vi "All.vi"() -> ()   [LabVIEW 2020]
uses:
  <vilib>/vision/driver/IMAQdx.llb/IMAQdx Buffer Number Mode.ctl
  <vilib>/vision/driver/NI_Vision_Acquisition_Software.lvlib
  <resource>/objmgr/imaqdx.rc
panel:
  out "data out":string
  out "y":dbl
  out "x":dbl
  in  "Server Closed":string="The server VI closed the connection."
  in  "Number of Images":u32=10
  in  "Camera Name":refnum<k21> caption="IMAQdx Session"
  in  "Stop":bool
  out "Processing Frame Rate":dbl
  out "Images Missed":u32
  out "Start Image":T1(plugin-control)
  out "Threshold  Image":T1(plugin-control)
  out "Fill Holes  Image":T1(plugin-control)
  in  "Green":cluster{"Lower value":i32, "Upper value":i32}={"Lower value"=168, "Upper value"=255} {"Lower value" scale=0.0..255.0; "Upper value" scale=0.0..255.0}
  in  "Blue":cluster{"Lower value":i32, "Upper value":i32}={"Lower value"=148, "Upper value"=255} {"Lower value" scale=0.0..255.0; "Upper value" scale=0.0..255.0}
  in  "Red":cluster{"Lower value":i32, "Upper value":i32}={"Lower value"=158, "Upper value"=255} {"Lower value" scale=0.0..255.0; "Upper value" scale=0.0..255.0}
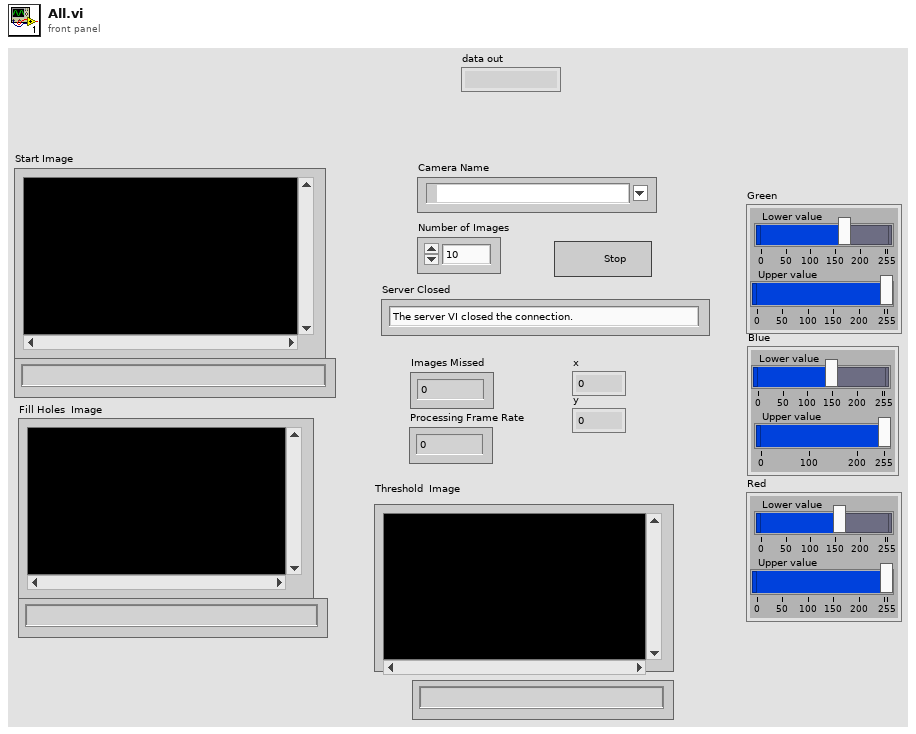
[diagram p1: front panel]
types:
  T1 = typedef "IMAQ Image.ctl" = refnum<image>
  T2 = typedef "IMAQdx.ctl" = refnum<k21>
  T3 = typedef "NI_Vision_Acquisition_Software.lvlib/IMAQdx Buffer Number Mode.ctl" = enum32{"Next", "Last", "Buffer Number", "Every", "Last New"}
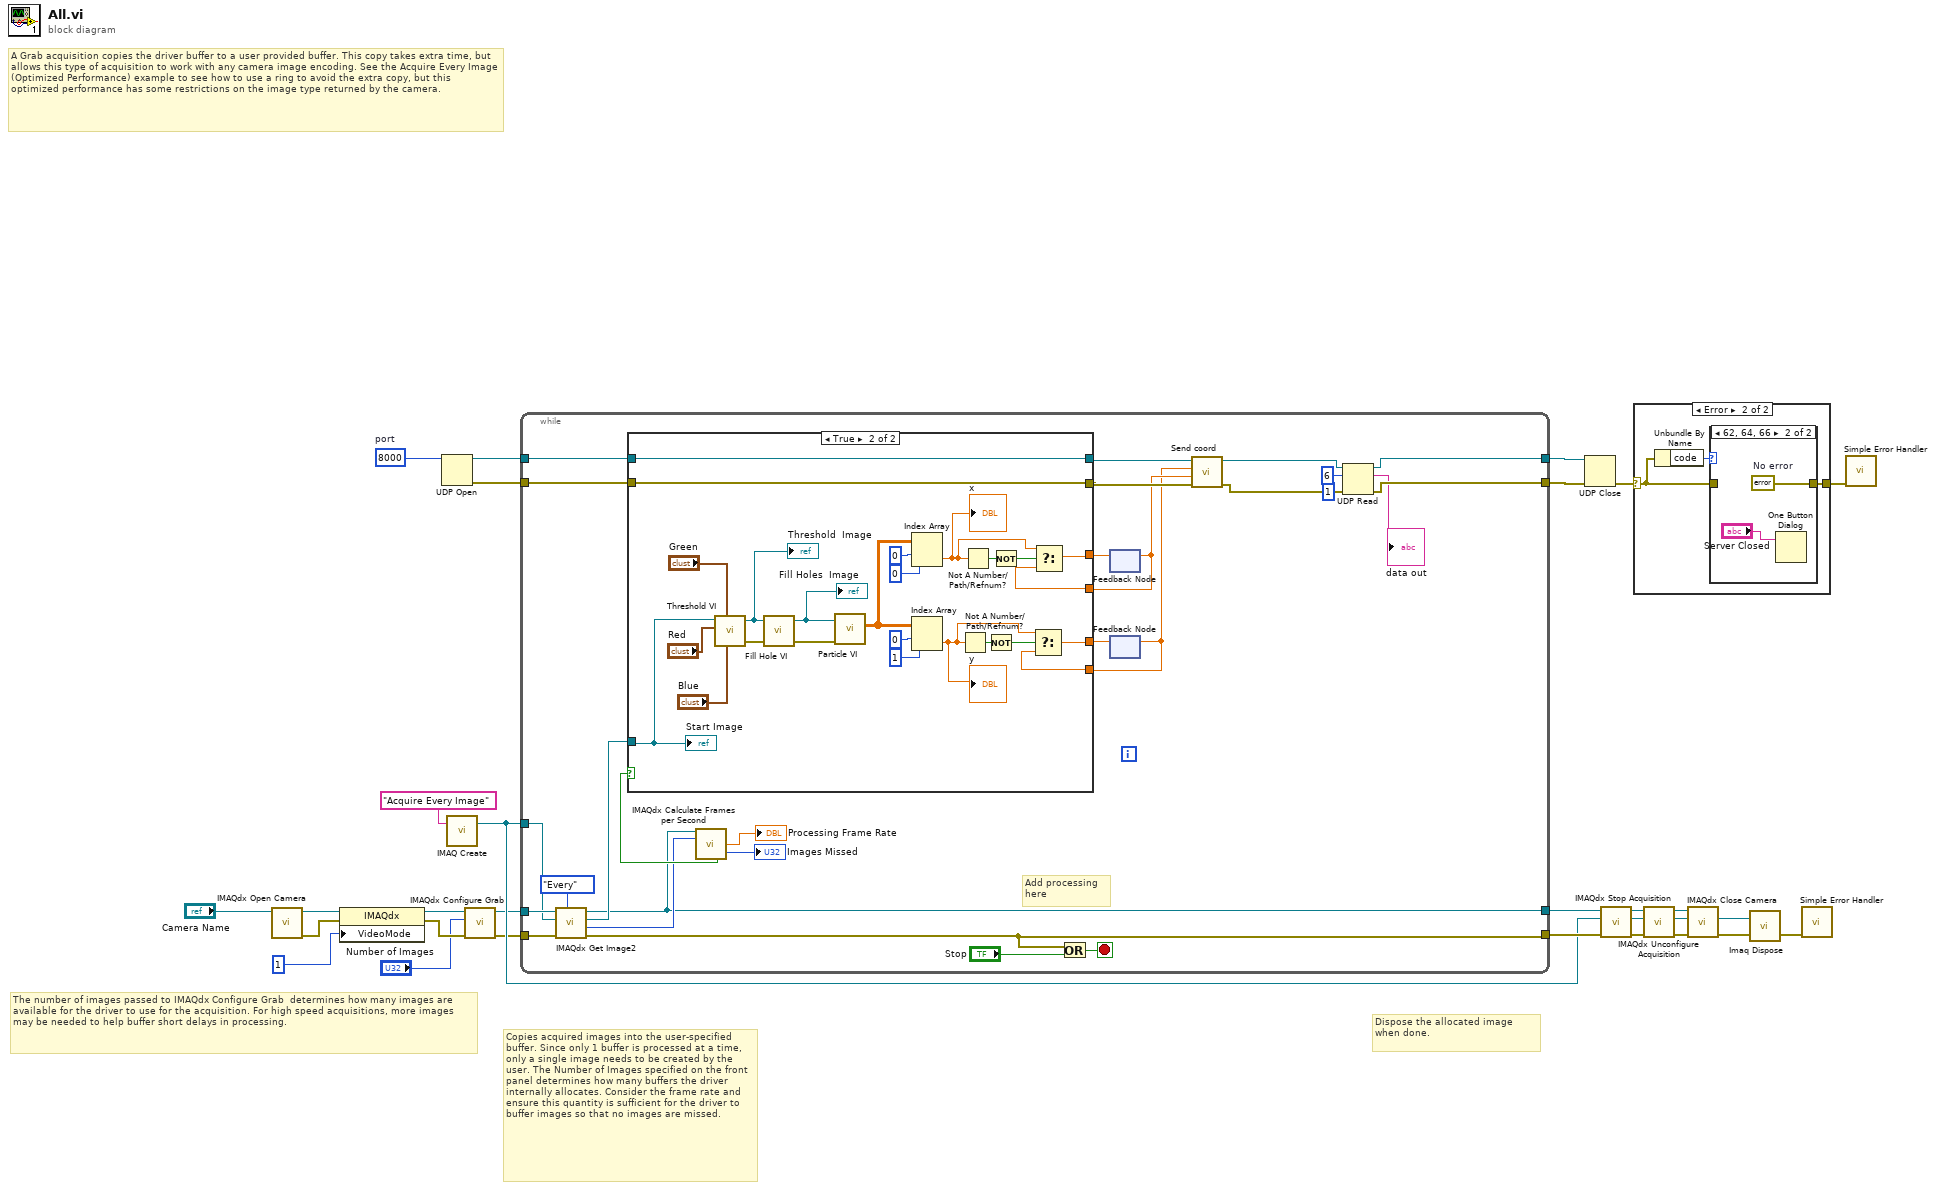
[diagram p0: block diagram]
diagram:
  w1 = u16 8000  # port
  # "The number of images passed to IMAQdx Configure Grab  determines how many images are available for the driver to use for the acquisition. For high speed acquisitions, more images may be needed to help buffer short delays in processing."
  # "Dispose the allocated image when done."
  # "A Grab acquisition copies the driver buffer to a user provided buffer. This copy takes extra time, but allows this type of acquisition to work with any camera image encoding. See the Acquire Every Image (Optimized Performance) example to see how to use a ring to avoid the extra copy, but this optimized performance has some restrictions on the image type returned by the camera."
  # "Copies acquired images into the user-specified buffer. Since only 1 buffer is processed at a time, only a single image needs to be created by the user. The Number of Images specified on the front panel determines how many buffers the driver internally allocates. Consider the frame rate and ensure this quantity is sufficient for the driver to buffer images so that no images are missed."
  n1 = call <vilib>:"IMAQdx Open Camera.vi"("Session In"="Camera Name") -> ("error out"=w18:errorcluster, "Session Out"=w19:T2)  [unwired: 2 in, 7 out]
  n2 = property class="IMAQdx"(reference=w19, error in=w18, "VideoMode"=u32 1) -> (reference out=w11:T2, error out=w10:errorcluster)
  n3 = UDP Open(11:w1) -> (port=w8:refnum<k16>, 0:w7:errorcluster)  [unwired: 4 in, 1 out]
  n4 = call "IMAQ Create"("Image Name"="Acquire Every Image") -> ("New Image"=w14:T1)  [unwired: 3 in, 2 out]
  n5 = call <vilib>:"IMAQdx Configure Grab.vi"("error in"=w10, "Number of Buffers"="Number of Images", "Session In"=w11) -> ("error out"=w12:errorcluster, "Session Out"=w13:T2)  [unwired: 7 in]
  n6 = while {
    tunnel: [w45] -> w16
    tunnel: w12 -> [w51]
    tunnel: w13 -> [w50]
    tunnel: [w34] -> w15
    tunnel: w14 -> [w48]
    tunnel: w8 -> [w43]
    tunnel: w7 -> [w42]
    tunnel: [w28] -> w4
    tunnel: [w29] -> w3
    stop <- w35 stop-if-true
    # "Avoid image display when falling behind."
    # "Add processing here"
    n7 = call <vilib>:"IMAQdx Get Image2.vi"("Buffer Number Mode (Next)"=IMAQdx_Buffer_Number_Mode."Every" ("Buffer Number Mode"), "error in"=w51, "Image In"=w48, "Session In"=w50) -> ("error out"=w34:errorcluster, "Buffer Number Out"=w47:u32, "Image Out"=w46:T1, "Session Out"=w45:T2)  [unwired: 4 in]
    n8 = call <vilib>:"IMAQdx Calculate Frames per Second.vi"("Session In"=w45, "Buffer Number"=w47) -> ("Update Display"=w52:bool, "Processed Frames per Second"=→"Processing Frame Rate":dbl, "Images Missed"=→"Images Missed":u32)  [unwired: 7 in, 4 out]
    n9 = Or(x=w34, y="Stop") -> (x .or. y?=w35:bool)
    n10 = feedback #1() -> (w38:dbl)  [unwired: 1 in]
    n11 = feedback #2() -> (w36:dbl)  [unwired: 1 in]
    n12 = case shown="True" w52 {
      tunnel: w46 -> [_ w77]
      tunnel: w43 -> [w58 w74]
      tunnel: w42 -> [w57 w76]
      tunnel: [w58 w74] -> w41
      tunnel: [w57 w76] -> w40
      tunnel: [w55 w67] -> w37
      tunnel: [w56 w68] -> w39
      tunnel: w38 -> [w56 w65]
      tunnel: w36 -> [w55 w66]
      frame False {
      }
      frame True {
        n13 = call "Threshold VI.vi"("Image In"=w77, "Green or Sat Range"="Green", "Red or Hue Range"="Red", "Blue or Luma or Val or Inten Range"="Blue") -> ("Image"=w75:T1, "error out"=w81:errorcluster)  [unwired: 3 in]
        "Threshold  Image" <- w75
        n14 = call "Fill Hole VI.vi"("error in (no error)"=w81, "Image In"=w75) -> ("error out"=w83:errorcluster, "Fill holes\nimage"=w82:T1)  [unwired: 2 in]
        "Fill Holes  Image" <- w82
        n15 = call "Particle VI.vi"("error in (no error)"=w83, "Image In"=w82) -> ("Particle Measurements (Pixels) (Particle Analysis 1)"=w69:dbl[][])  [unwired: 1 in, 4 out]
        n16 = Index Array(array=w69, index (row)=0, index (col)=0) -> (element=w64:dbl)
        "x" <- w64
        n17 = Index Array(array=w69, index (row)=0, index (col)=1) -> (element=w59:dbl)
        "y" <- w59
        n18 = Not A Number/Path/Refnum?(number/path/refnum=w59) -> (NaN/Path/Refnum?=w61:bool)
        n19 = Not A Number/Path/Refnum?(number/path/refnum=w64) -> (NaN/Path/Refnum?=w63:bool)
        n20 = Not(x=w61) -> (.not. x?=w60:bool)
        n21 = Not(x=w63) -> (.not. x?=w62:bool)
        n22 = Select(t=w59, s=w60, f=w66) -> (s? t:f=w67:dbl)
        n23 = Select(t=w64, s=w62, f=w65) -> (s? t:f=w68:dbl)
        "Start Image" <- w77
      }
    }
    n24 = feedback-in #1(w39) -> ()
    n25 = feedback-in #2(w37) -> ()
    n26 = call "Send coord.vi"("error in (no error)"=w40, "x"=w38, "y"=w36, "connection ID"=w41) -> ("error out"=w32:errorcluster, "connection ID out"=w33:refnum<k16>)  [unwired: 6 in]
    n27 = UDP Read(connection ID=w33, max size (548)=6, timeout ms (25000)=1, 8:w32) -> (data out=→"data out":string, error out=w28:errorcluster, 3:w29:refnum<k16>)  [unwired: 2 out]
  }
  n28 = UDP Close(connection ID=w3, 8:w4) -> (error out=w6:errorcluster)  [unwired: 1 out]
  n29 = call <vilib>:"IMAQdx Stop Acquisition.vi"("error in"=w15, "Session In"=w16) -> ("error out"=w22:errorcluster, "Session Out"=w23:T2)  [unwired: 8 out]
  n30 = case shown="Error" w6 {
    selector: w6 -> [w84 w86]
    tunnel: [w84 w85] -> w5
    frame No Error {
    }
    frame Error {
      n31 = Unbundle By Name(w86) -> ("code"=w87:i32)
      n32 = case shown="62, 64, 66" w87 {
        tunnel: w86 -> [w88 _]
        tunnel: [w88 w90] -> w85
        frame Default {
        }
        frame 62, 64, 66 {
          w90 = errorcluster {"status"=FALSE, "code"=0, "source"=""}  # No error
          n33 = One Button Dialog(message="Server Closed") -> ()  [unwired: 1 in, 1 out]
        }
      }
    }
  }
  n34 = call <vilib>:"IMAQdx Unconfigure Acquisition.vi"("error in"=w22, "Session In"=w23) -> ("error out"=w25:errorcluster, "Session Out"=w24:T2)  [unwired: 8 out]
  n35 = call <vilib>:"IMAQdx Close Camera.vi"("error in"=w25, "Session In"=w24) -> ("error out"=w21:errorcluster)  [unwired: 9 out]
  n36 = call "Imaq Dispose"("Image"=w14, "error in (no error)"=w21) -> ("error out"=w20:errorcluster)  [unwired: 4 in]
  n37 = call <vilib>:"Simple Error Handler.vi"("error in (no error)"=w20) -> ()  [unwired: 4 in, 5 out]
  n38 = call <vilib>:"Simple Error Handler.vi"("error in (no error)"=w5) -> ()  [unwired: 4 in, 5 out]
